vi "Auto Further Switch.vi"() -> ()   [LabVIEW 2017]
uses:
  LabVIEW_is_Under_Control.lib/Util/Unpack Gamepad/Button Cluster.ctl
  Team Code/Robot Global Data.vi
panel:
  in  "Time to wait (min 50ms) 3":dbl=50.0
  in  "Delay Fwd 3":i32=500
  in  "DistanceSwitch 3":dbl=400.0
  in  "Delay Turn 2":i32=200
  in  "Turn 2":dbl=-90.0 format="%#_13g"
  in  "Delay Fwd 2":i32=200
  in  "DistanceAfterTurn":dbl=40.0
  in  "Right?":bool
  in  "Delay Turn":i32=200
  in  "Turn":dbl=-90.0 format="%#_13g"
  in  "Delay Fwd":i32=500
  in  "DistanceFwd":dbl=400.0
  in  "Time to wait (min 50ms)":dbl=50.0
  in  "Time to wait (min 50ms) 2":dbl=50.0
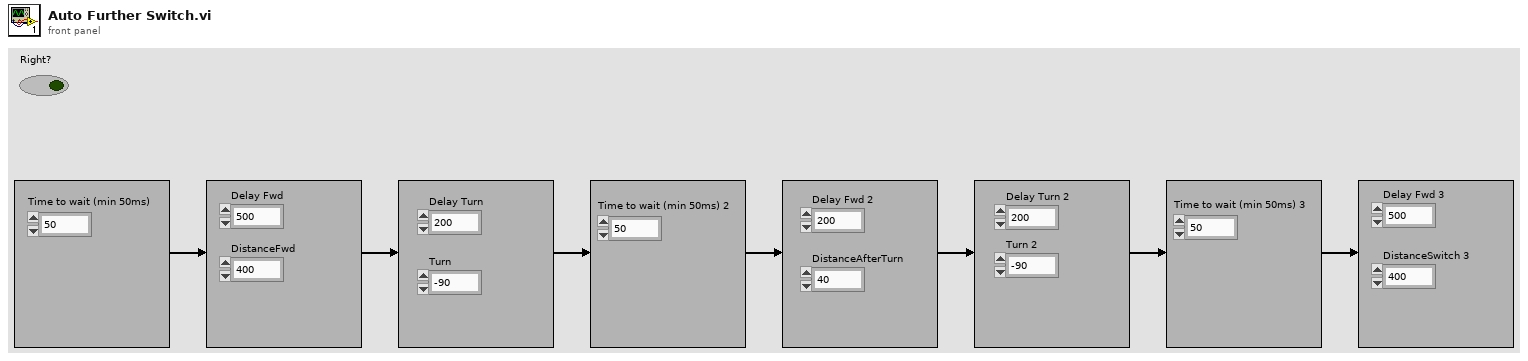
[diagram p1: front panel]
types:
  T1 = enum16{"Zerandosensor", "Andando", "Girando", "Zerandosensor2", "Andando2", "Girando2", "Zerandosensor3", "Andando3", "Score", "Finalizando"}
  T2 = typedef "Button Cluster.ctl" = cluster{"Buttons[0]":bool, "Buttons[1]":bool, "Buttons[2]":bool, "Buttons[3]":bool, "Buttons[4]":bool, "Buttons[5]":bool, "Buttons[6]":bool, "Buttons[7]":bool, "Buttons[8]":bool, "Buttons[9]":bool}
  T3 = cluster{"proportional gain (Kc)":dbl, "integral time (Ti, min)":dbl, "derivative time (Td, min)":dbl}
  T4 = enum16{"Zerandosensor", "Andando", "Girando", "Zerandosensor2", "Andando2", "Girando2", "Zerandosensor3", "Andando3", "Score", "Finalizando", "Jogando"}
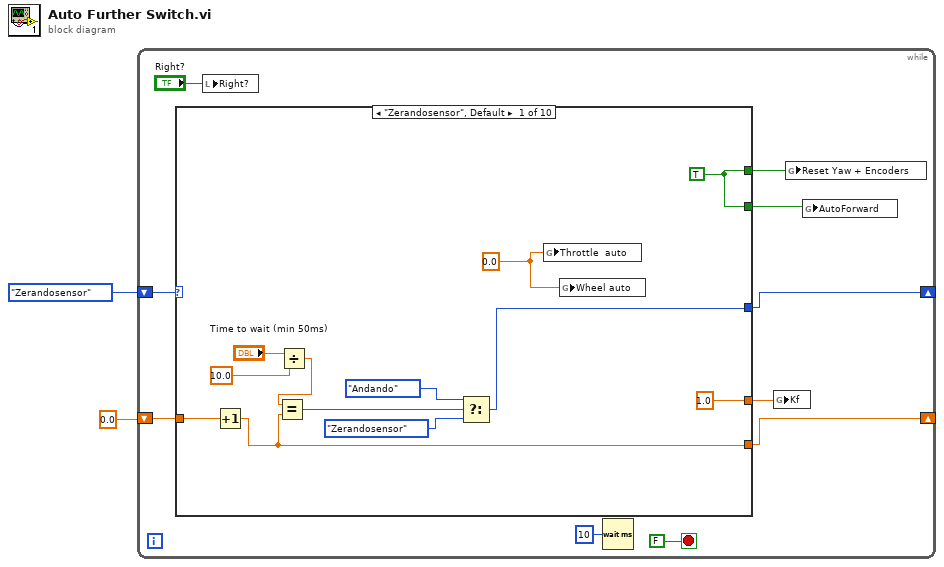
[diagram p0: block diagram]
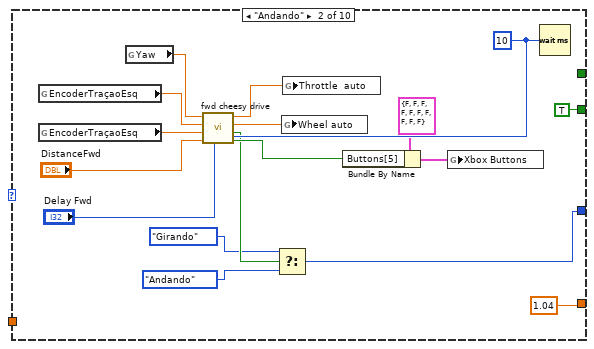
[diagram p2: hidden frame]
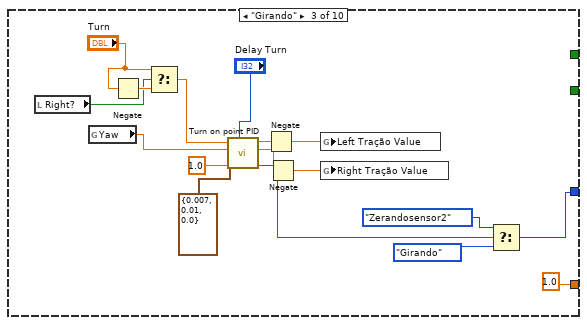
[diagram p3: hidden frame]
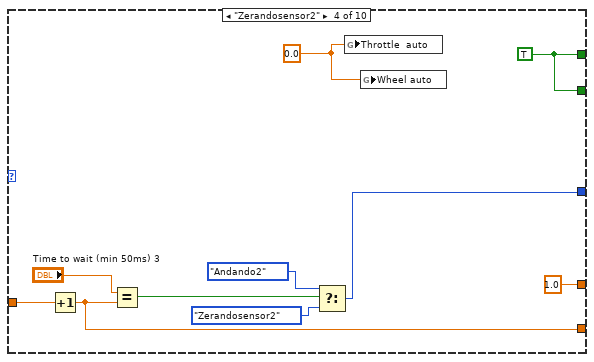
[diagram p4: hidden frame]
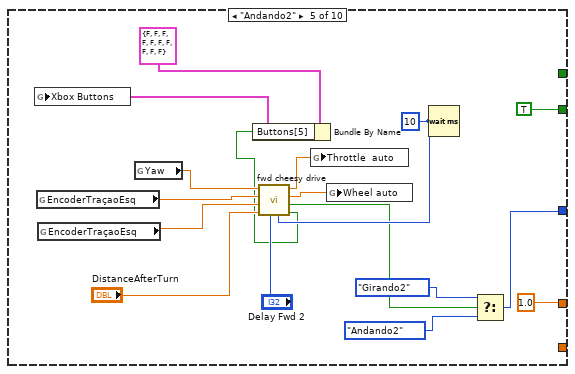
[diagram p5: hidden frame]
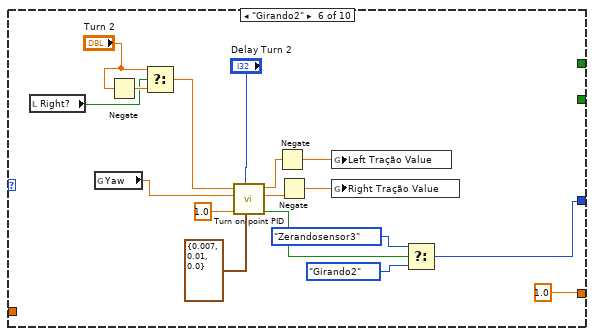
[diagram p6: hidden frame]
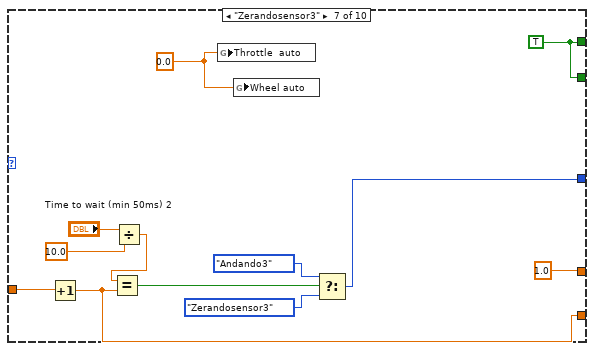
[diagram p7: hidden frame]
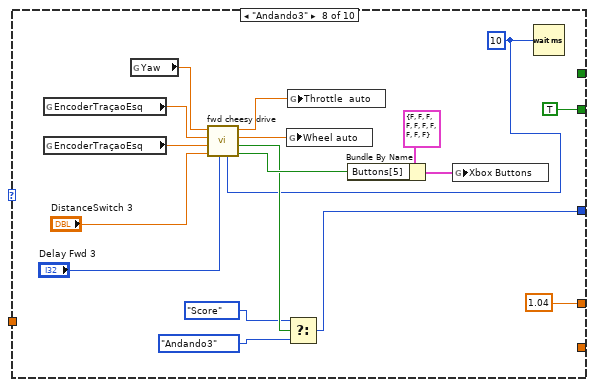
[diagram p8: hidden frame]
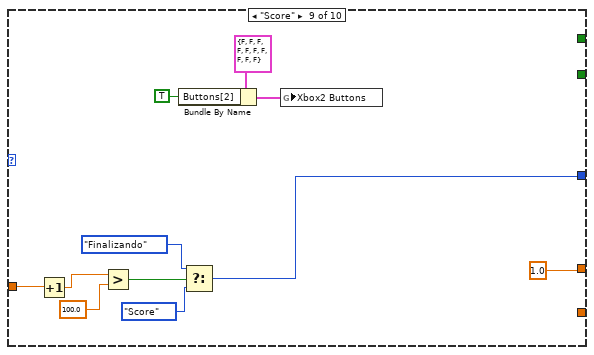
[diagram p9: hidden frame]
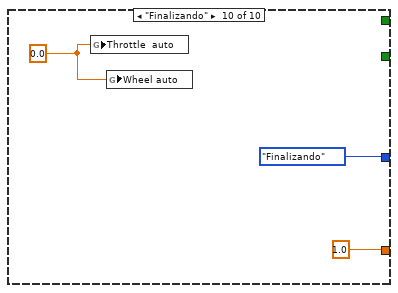
[diagram p10: hidden frame]
diagram:
  n1 = while {
    shift-right: [w4] -> _
    shift-left: T1."Zerandosensor" -> [w3]
    shift-right: [w6] -> _
    shift-left: 0.0 -> [w7]
    stop <- FALSE stop-if-true
    n2 = case shown="\"Zerandosensor\", Default" w3 {
      tunnel: [w24 _ _ w66 _ _ w106 _ _ _] -> w9
      tunnel: [w24 TRUE _ w66 TRUE _ w106 TRUE _ _] -> w10
      tunnel: [1.0 1.04 1.0 1.0 1.0 1.0 1.0 1.04 1.0 1.0] -> w8
      tunnel: w7 -> [w20 _ _ w64 _ _ w111 _ w142 _]
      tunnel: [w19 _ _ w63 _ _ w108 _ _ _] -> w6
      tunnel: [w15 w27 w45 w62 w71 w89 w105 w117 w135 T4."Finalizando"] -> w4
      frame "Zerandosensor", Default {
        w16 = 0.0
        w24 = TRUE
        n3 = Increment(x=w20) -> (x+1=w19:dbl)
        n4 = Divide(x="Time to wait (min 50ms)", y=10.0) -> (x/y=w18:dbl)
        n5 = Equal?(x=w18, y=w19) -> (x = y?=w17:bool)
        n6 = Select(t=T1."Andando", s=w17, f=T1."Zerandosensor") -> (s? t:f=w15:T1)
        n7 = global write "Robot Global Data.vi" "Throttle  auto"(w16) -> ()
        n8 = global write "Robot Global Data.vi" "Wheel auto"(w16) -> ()
      }
      frame "Andando" {
        w35 = u32 10 ("milliseconds to wait")
        n9 = global read "Robot Global Data.vi" "EncoderTraçaoEsq"() -> (w37:dbl)
        n10 = global read "Robot Global Data.vi" "EncoderTraçaoEsq"() -> (w38:dbl)
        n11 = global read "Robot Global Data.vi" "Yaw"() -> (w39:dbl)
        n12 = call "fwd cheesy drive.vi"("Loop Timer"=w35, "Time to stop"="Delay Fwd", "Distance"="DistanceFwd", "Encoder Left"=w38, "Encoder Right"=w37, "Yaw"=w39) -> ("Finished distance"=w30:bool, "Both finished"=w29:bool, "Direction"=w34:dbl, "Trottle"=w33:dbl)  [unwired: 2 in]
        n13 = Select(t=T1."Girando", s=w29, f=T1."Andando") -> (s? t:f=w27:T1)
        n14 = global write "Robot Global Data.vi" "Wheel auto"(w34) -> ()
        n15 = global write "Robot Global Data.vi" "Throttle  auto"(w33) -> ()
        n16 = Bundle By Name(cluster=T2 {"Buttons[0]"=FALSE, "Buttons[1]"=FALSE, "Buttons[2]"=FALSE, "Buttons[3]"=FALSE, "Buttons[4]"=FALSE, "Buttons[5]"=FALSE, "Buttons[6]"=FALSE, "Buttons[7]"=FALSE, "Buttons[8]"=FALSE, "Buttons[9]"=FALSE} ("Xbox Buttons"), "Buttons[5]"=w30) -> (w31:T2)
        n17 = global write "Robot Global Data.vi" "Xbox Buttons"(w31) -> ()
        n18 = Wait (ms)(milliseconds to wait=w35) -> ()  [unwired: 1 out]
      }
      frame "Girando" {
        n19 = local read "Right?"() -> (w44:bool)
        n20 = global read "Robot Global Data.vi" "Yaw"() -> (w51:dbl)
        n21 = Negate(x="Turn") -> (-x=w48:dbl)
        n22 = Select(t="Turn", s=w44, f=w48) -> (s? t:f=w46:dbl)
        n23 = call "Turn on point PID.vi"("Gains"=T3 {"proportional gain (Kc)"=0.007, "integral time (Ti, min)"=0.01, "derivative time (Td, min)"=0.0}, "Time to stop"="Delay Turn", "Precision"=1.0, "Yaw"=w51, "Setpoint(degrees)"=w46) -> ("Finished?"=w56:bool, "PWM right"=w52:dbl, "PWM left"=w53:dbl)  [unwired: 4 in]
        n24 = Negate(x=w53) -> (-x=w50:dbl)
        n25 = Negate(x=w52) -> (-x=w49:dbl)
        n26 = global write "Robot Global Data.vi" "Left Tração Value"(w50) -> ()
        n27 = global write "Robot Global Data.vi" "Right Tração Value"(w49) -> ()
        n28 = Select(t=T1."Zerandosensor2", s=w56, f=T1."Girando") -> (s? t:f=w45:T1)
      }
      frame "Zerandosensor2" {
        w68 = 0.0
        w66 = TRUE
        n29 = Increment(x=w64) -> (x+1=w63:dbl)
        n30 = Equal?(x="Time to wait (min 50ms) 3", y=w63) -> (x = y?=w65:bool)
        n31 = Select(t=T1."Andando2", s=w65, f=T1."Zerandosensor2") -> (s? t:f=w62:T1)
        n32 = global write "Robot Global Data.vi" "Throttle  auto"(w68) -> ()
        n33 = global write "Robot Global Data.vi" "Wheel auto"(w68) -> ()
      }
      frame "Andando2" {
        w79 = u32 10 ("milliseconds to wait")
        n34 = global read "Robot Global Data.vi" "EncoderTraçaoEsq"() -> (w81:dbl)
        n35 = global read "Robot Global Data.vi" "EncoderTraçaoEsq"() -> (w82:dbl)
        n36 = global read "Robot Global Data.vi" "Yaw"() -> (w83:dbl)
        n37 = call "fwd cheesy drive.vi"("Loop Timer"=w79, "Time to stop"="Delay Fwd 2", "Distance"="DistanceAfterTurn", "Encoder Left"=w82, "Encoder Right"=w81, "Yaw"=w83) -> ("Finished distance"=w73:bool, "Both finished"=w72:bool, "Direction"=w77:dbl, "Trottle"=w76:dbl)  [unwired: 2 in]
        n38 = Bundle By Name(cluster=T2 {"Buttons[0]"=FALSE, "Buttons[1]"=FALSE, "Buttons[2]"=FALSE, "Buttons[3]"=FALSE, "Buttons[4]"=FALSE, "Buttons[5]"=FALSE, "Buttons[6]"=FALSE, "Buttons[7]"=FALSE, "Buttons[8]"=FALSE, "Buttons[9]"=FALSE} ("Xbox Buttons"), "Buttons[5]"=w73) -> (w74:T2)
        n39 = global write "Robot Global Data.vi" "Xbox Buttons"(w74) -> ()
        n40 = global write "Robot Global Data.vi" "Throttle  auto"(w76) -> ()
        n41 = global write "Robot Global Data.vi" "Wheel auto"(w77) -> ()
        n42 = Wait (ms)(milliseconds to wait=w79) -> ()  [unwired: 1 out]
        n43 = Select(t=T1."Girando2", s=w72, f=T1."Andando2") -> (s? t:f=w71:T1)
      }
      frame "Girando2" {
        n44 = local read "Right?"() -> (w88:bool)
        n45 = global read "Robot Global Data.vi" "Yaw"() -> (w95:dbl)
        n46 = Negate(x="Turn 2") -> (-x=w92:dbl)
        n47 = Select(t="Turn 2", s=w88, f=w92) -> (s? t:f=w90:dbl)
        n48 = call "Turn on point PID.vi"("Gains"=T3 {"proportional gain (Kc)"=0.007, "integral time (Ti, min)"=0.01, "derivative time (Td, min)"=0.0}, "Time to stop"="Delay Turn 2", "Precision"=1.0, "Yaw"=w95, "Setpoint(degrees)"=w90) -> ("Finished?"=w100:bool, "PWM right"=w96:dbl, "PWM left"=w97:dbl)  [unwired: 4 in]
        n49 = Negate(x=w97) -> (-x=w94:dbl)
        n50 = Negate(x=w96) -> (-x=w93:dbl)
        n51 = global write "Robot Global Data.vi" "Left Tração Value"(w94) -> ()
        n52 = global write "Robot Global Data.vi" "Right Tração Value"(w93) -> ()
        n53 = Select(t=T1."Zerandosensor3", s=w100, f=T1."Girando2") -> (s? t:f=w89:T1)
      }
      frame "Zerandosensor3" {
        w106 = TRUE
        w109 = 0.0
        n54 = Increment(x=w111) -> (x+1=w108:dbl)
        n55 = Divide(x="Time to wait (min 50ms) 2", y=10.0) -> (x/y=w112:dbl)
        n56 = Equal?(x=w112, y=w108) -> (x = y?=w110:bool)
        n57 = global write "Robot Global Data.vi" "Throttle  auto"(w109) -> ()
        n58 = global write "Robot Global Data.vi" "Wheel auto"(w109) -> ()
        n59 = Select(t=T1."Andando3", s=w110, f=T1."Zerandosensor3") -> (s? t:f=w105:T1)
      }
      frame "Andando3" {
        w118 = u32 10 ("milliseconds to wait")
        n60 = global read "Robot Global Data.vi" "EncoderTraçaoEsq"() -> (w127:dbl)
        n61 = global read "Robot Global Data.vi" "EncoderTraçaoEsq"() -> (w128:dbl)
        n62 = global read "Robot Global Data.vi" "Yaw"() -> (w129:dbl)
        n63 = call "fwd cheesy drive.vi"("Loop Timer"=w118, "Time to stop"="Delay Fwd 3", "Distance"="DistanceSwitch 3", "Encoder Left"=w128, "Encoder Right"=w127, "Yaw"=w129) -> ("Finished distance"=w120:bool, "Both finished"=w119:bool, "Direction"=w124:dbl, "Trottle"=w123:dbl)  [unwired: 2 in]
        n64 = global write "Robot Global Data.vi" "Wheel auto"(w124) -> ()
        n65 = global write "Robot Global Data.vi" "Throttle  auto"(w123) -> ()
        n66 = Select(t=T1."Score", s=w119, f=T1."Andando3") -> (s? t:f=w117:T1)
        n67 = Bundle By Name(cluster=T2 {"Buttons[0]"=FALSE, "Buttons[1]"=FALSE, "Buttons[2]"=FALSE, "Buttons[3]"=FALSE, "Buttons[4]"=FALSE, "Buttons[5]"=FALSE, "Buttons[6]"=FALSE, "Buttons[7]"=FALSE, "Buttons[8]"=FALSE, "Buttons[9]"=FALSE} ("Xbox Buttons"), "Buttons[5]"=w120) -> (w121:T2)
        n68 = global write "Robot Global Data.vi" "Xbox Buttons"(w121) -> ()
        n69 = Wait (ms)(milliseconds to wait=w118) -> ()  [unwired: 1 out]
      }
      frame "Score" {
        n70 = Increment(x=w142) -> (x+1=w141:dbl)
        n71 = Greater?(x=w141, y=100.0) -> (0:w139:bool)
        n72 = Bundle By Name(cluster=T2 {"Buttons[0]"=FALSE, "Buttons[1]"=FALSE, "Buttons[2]"=FALSE, "Buttons[3]"=FALSE, "Buttons[4]"=FALSE, "Buttons[5]"=FALSE, "Buttons[6]"=FALSE, "Buttons[7]"=FALSE, "Buttons[8]"=FALSE, "Buttons[9]"=FALSE} ("Xbox Buttons"), "Buttons[2]"=TRUE) -> (w133:T2)
        n73 = Select(t=T4."Finalizando", s=w139, f=T4."Score") -> (s? t:f=w135:T4)
        n74 = global write "Robot Global Data.vi" "Xbox2 Buttons"(w133) -> ()
      }
      frame "Finalizando" {
        w145 = 0.0
        n75 = global write "Robot Global Data.vi" "Throttle  auto"(w145) -> ()
        n76 = global write "Robot Global Data.vi" "Wheel auto"(w145) -> ()
      }
    }
    n77 = local write "Right?"("Right?") -> ()
    n78 = Wait (ms)(milliseconds to wait=u32 10) -> ()  [unwired: 1 out]
    n79 = global write "Robot Global Data.vi" "Kf"(w8) -> ()
    n80 = global write "Robot Global Data.vi" "Reset Yaw + Encoders"(w9) -> ()
    n81 = global write "Robot Global Data.vi" "AutoForward"(w10) -> ()
  }
